vi "Variant Cluster Create.vi"(8 "error in (no error)":errorcluster, 11 "Elements":variant[](array[variant])) -> (0 "error out":errorcluster, 3 "Cluster":variant)   [LabVIEW 2018, in "labview_json.lvlib"]
uses:
  labview_json.lvlib
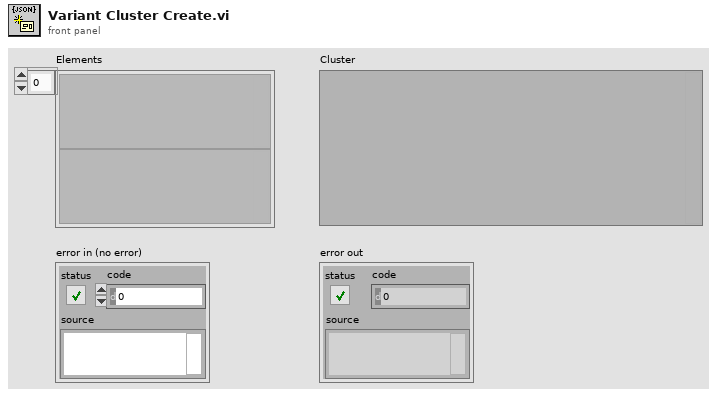
[diagram p1: front panel]
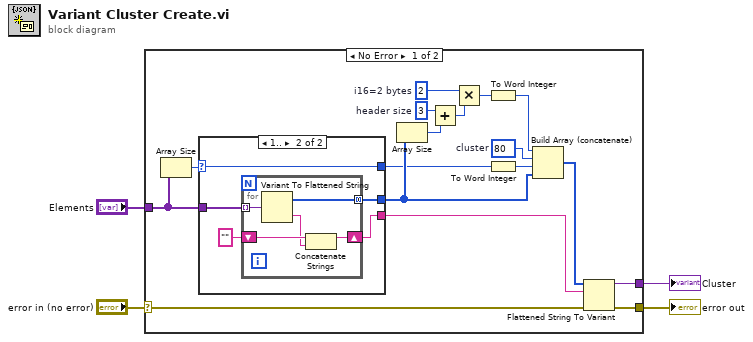
[diagram p0: block diagram]
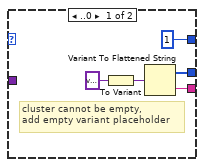
[diagram p2: hidden frame]
diagram:
  n1 = case shown="No Error" "error in (no error)" {
    selector: "error in (no error)" -> [w19 w37]
    tunnel: "Elements" -> [w20 _]
    tunnel: [w18 w37] -> w2
    tunnel: [w17 _] -> w1
    frame No Error {
      w10 = i16 80  # cluster
      w14 = 2  # i16=2 bytes
      w15 = 3  # header size
      n2 = Array Size(array=w20) -> (size(s)=w21:i32)
      n3 = case shown="1.." w21 {
        selector: w21 -> [_ w31]
        tunnel: w20 -> [_ w30]
        tunnel: [1 w31] -> w5
        tunnel: [w24 w29] -> w8
        tunnel: [w23 w27] -> w7
        frame ..0 {
          # "cluster cannot be empty,\nadd empty variant placeholder"
          n4 = To Variant(anything=variant) -> (Variant=w26:variant)
          n5 = Variant To Flattened String(Variant=w26) -> (data string=w23:string, 1:w24:i16[])
        }
        frame 1.. {
          n6 = for {
            tunnel: w30 -> [w36] mode=indexing
            tunnel: [w35] -> w29 mode=concatenating
            shift-right: [w32] -> w27
            shift-left: "" -> [w34]
            n7 = Variant To Flattened String(Variant=w36) -> (data string=w33:string, 1:w35:i16[])
            n8 = Concatenate Strings(w34, w33) -> (w32:string)
          }
        }
      }
      n9 = Array Size(array=w8) -> (size(s)=w6:i32)
      n10 = Add(x=w15, y=w6) -> (x+y=w13:i32)
      n11 = Multiply(x=w14, y=w13) -> (x*y=w12:i32)
      n12 = To Word Integer(number=w12) -> (16bit integer=w11:i16)
      n13 = To Word Integer(number=w5) -> (16bit integer=w9:i16)
      n14 = Build Array (concatenate)(w11, w10, w9, w8) -> (w16:i16[])
      n15 = Flattened String To Variant(4:w19, 6:w7, 7:w16) -> (0:w18:errorcluster, 3:w17:variant)
    }
    frame Error {
    }
  }
  "error out" <- w2
  "Cluster" <- w1
